vi "Actor Core.vi"(8 "error in":errorcluster, 11 "WebSocket Connection in":refnum<class "WebSocket Connection.lvclass">) -> (0 "error out":errorcluster, 3 "Actor out":refnum<class "Actor.lvclass">)   [LabVIEW 2021, in "WebSocket Actors.lvlib" / "WebSocket Connection.lvclass"]
doc: "(<B>Filename</B>: Actor Framework.lvlib:Actor.lvclass:Actor Core.vi)\n\nReceives messages to the actor, reacts to them, and initiates any error handling that may shut the actor down.\n\nDescendant classes may override this VI to append parallel tasks for the actor to complete while it handles messages. Overrides use the Call Parent Method node."
uses:
  WebSocket Connection.lvclass
  C:/Program Files/National Instruments/LabVIEW 2021/vi.lib/ActorFramework/Actor/Actor.lvclass
  <vilib>/ActorFramework/Actor/Actor.lvclass
  Abstract Messages/WebSocket Connection Handler Msg/properties/Connection Event.ctl
  Abstract Messages/WebSocket Connection Handler Msg/typedefs/Message Data.ctl
  <vilib>/ActorFramework/Message Enqueuer/Message Enqueuer.lvclass
  <vilib>/LS Instruments AG/LV-WebSockets/Data Format.ctl
  <vilib>/ActorFramework/Actor/Actor.lvclass/Actor.ctl
  <vilib>/ActorFramework/Message Enqueuer/Message Enqueuer.lvclass/Message Enqueuer.ctl
  WebSocket Connection.lvclass/WebSocket Connection.ctl
  Abstract Messages/WebSocket Connection Handler Msg/WebSocket Connection Handler Msg.lvclass/WebSocket Connection Handler Msg.ctl
  Connection Status.ctl
  <vilib>/ActorFramework/Report Error Msg/Report Error Msg.lvclass/Report Error Msg.ctl
  <vilib>/ActorFramework/Message Enqueuer/Init from Existing Queue.vi
  <vilib>/ActorFramework/Message Enqueuer/Enqueue.vi
  <vilib>/GPower/Error/Library/SplitAppended.vi
  <vilib>/GPower/Error/Library/AppendErrors.vi
  <vilib>/GPower/Error/Library/Append/AppendMulti.vi
  <vilib>/GPower/Error/Library/SubVIs/ExplanationToError.vi
  <vilib>/dlg_ctls.llb/Space Constant.vi
  Abstract Messages/WebSocket Connection Handler Msg/WebSocket Connection Handler Msg.lvclass
  C:/Program Files/National Instruments/LabVIEW 2021/vi.lib/ActorFramework/Message/Message.lvclass
  <vilib>/ActorFramework/Report Error Msg/Report Error Msg.lvclass
  <vilib>/ActorFramework/Stop Msg/Stop Msg.lvclass
  <vilib>/Utility/LVClass/Get LV Class Name.vi
  <resource>/AFDebug/Generate Trace for Message.vi
  <vilib>/ActorFramework/Message Priority Queue/Priority Enqueue.vi
  <vilib>/Utility/error.llb/Error Cluster From Error Code.vi
  <vilib>/Utility/error.llb/Trim Whitespace.vi
  <vilib>/Utility/error.llb/Error Code Database.vi
  <vilib>/GPower/Error/Library/Append/AppendSingle.vi
  <vilib>/ErrorRing/Error Ring.xnode
  WebSocket Connection Messages/Write Connection Status Msg/Write Connection Status Msg.lvclass
  <vilib>/LS Instruments AG/LV-WebSockets/LV WebSockets.lvlib
  <vilib>/GPower/Error/GPError.lvlib
  C:/Projects/WebSocket-Actor/WebSocket Actor/WebSocket Connection/WebSocket Connection.lvclass
  Keepalive Heartbeat Messages/Report Pong Msg/Report Pong Msg.lvclass
  <userlib>/_OpenG.lib/error/error.llb/openg_error.lvlib
panel:
  out "Received Data":string
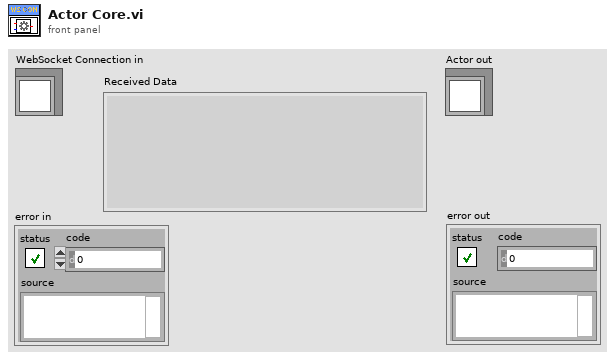
[diagram p1: front panel]
types:
  T1 = typedef "WebSocket Actors.lvlib/WebSocket Connection Handler Msg.lvclass/Message Data.ctl" = cluster{"Data":string, "Peer ID":string, "Connection Enqueuer":refnum<class "Message Enqueuer.lvclass">, "Data Format":T2}
  T2 = typedef "LV WebSockets.lvlib/Data Format.ctl" = enum16{"Text", "Binary"}
  T3 = typedef "WebSocket Actors.lvlib/WebSocket Connection Handler Msg.lvclass/Connection Event.ctl" = enum16{"On Connect", "On Message", "On Close", "On Drop"}
  T4 = typedef "WebSocket Actors.lvlib/WebSocket Connection.lvclass/Connection Status.ctl" = enum16{"Open", "Closed by Self", "Closed by Peer", "Dropped"}
  T5 = typedef "LV WebSockets.lvlib/Opcode.ctl" = enum8{"Continuation Frame", "Text Frame", "Binary Frame", "Reserved 3", "Reserved 4", "Reserved 5", "Reserved 6", "Reserved 7", "Connection Close", "Ping", "Pong", "Reserved B", "Reserved C", "Reserved D", "Reserved F"}
  T6 = typedef "LV WebSockets.lvlib/StatusCode.ctl" = u16
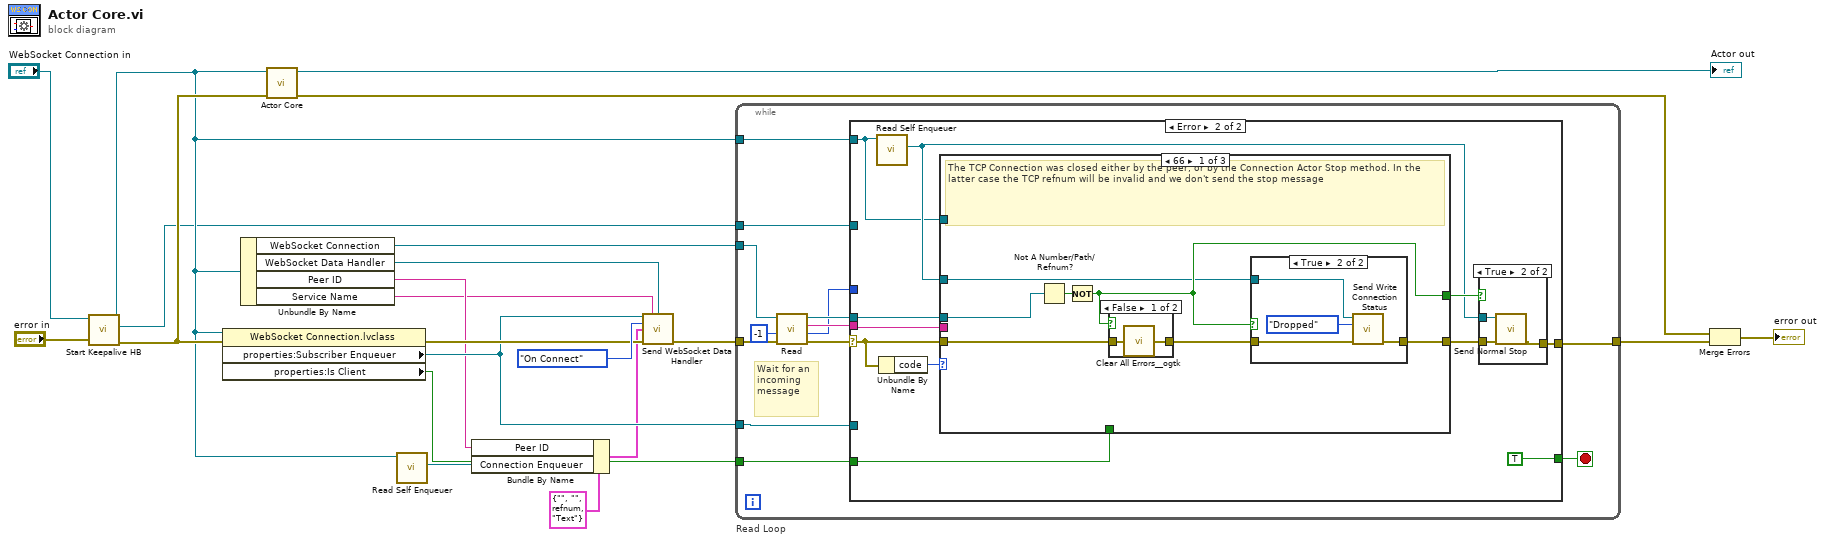
[diagram p0: block diagram]
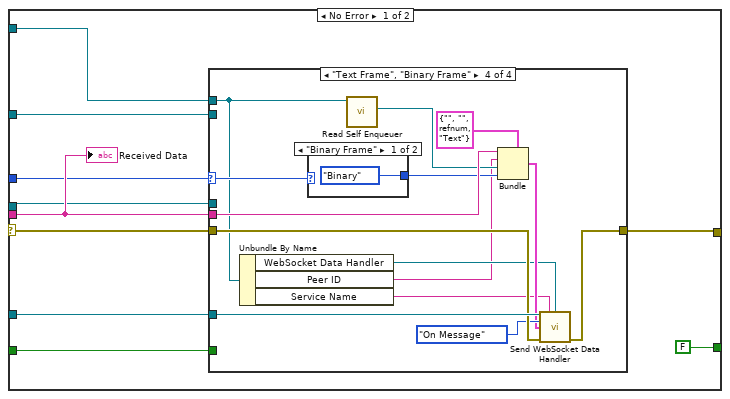
[diagram p2: hidden frame]
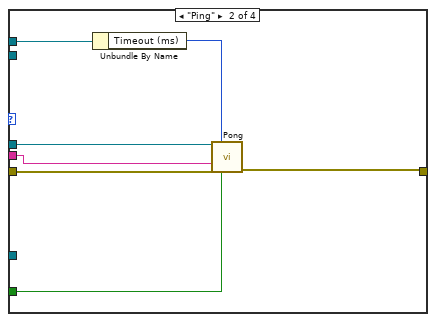
[diagram p4: hidden frame]
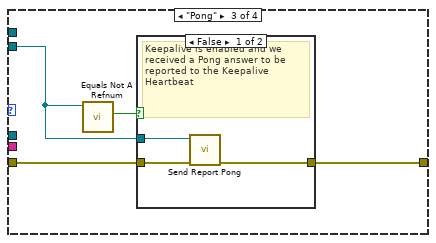
[diagram p5: hidden frame]
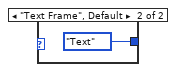
[diagram p7: hidden frame]
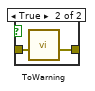
[diagram p10: hidden frame]
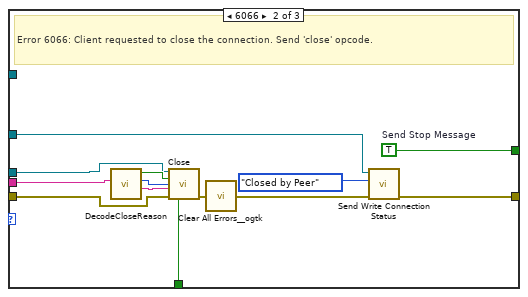
[diagram p11: hidden frame]
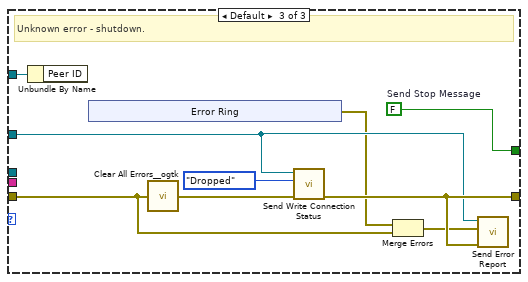
[diagram p12: hidden frame]
diagram:
  n1 = call "Start Keepalive HB.vi"("error in (no error)"="error in", "WebSocket Connection in"="WebSocket Connection in") -> ("error out"=w4:errorcluster, "Keepalive Heartbeat's Enqueuer"=w1:refnum<class "Message Enqueuer.lvclass">, "WebSocket Connection out"=w2:refnum<class "WebSocket Connection.lvclass">)  [unwired: 7 in]
  n2 = property class="WebSocket Connection.lvclass"(reference=w2, error in=w4) -> (error out=w13:errorcluster, "properties:Subscriber Enqueuer"=w12:refnum<class "Message Enqueuer.lvclass">, "properties:Is Client"=w11:bool)  [unwired: 1 out]
  n3 = Unbundle By Name(w2) -> ("WebSocket Connection"=w20:refnum<k5>, "WebSocket Data Handler"=w17:refnum<class "WebSocket Connection Handler Msg.lvclass">, "Peer ID"=w8:string, "Service Name"=w6:string)
  n4 = call-parent "Actor Core.vi"("error in"=w4, "Actor in"=w2) -> ("error out"=w21:errorcluster, "Actor out"=→"Actor out":refnum<class "Actor.lvclass">)  [unwired: 8 in]
  n5 = call <vilib>:"Read Self Enqueuer.vi"("Actor"=w2) -> ("Self Enqueuer"=w9:refnum<class "Message Enqueuer.lvclass">)  [unwired: 10 in]
  n6 = Bundle By Name(cluster=T1 {"Data"="", "Peer ID"="", "Connection Enqueuer"=refnum, "Data Format"=enum."Text"} ("Connection Message Data"), "Peer ID"=w8, "Connection Enqueuer"=w9) -> (w7:T1)
  n7 = call "Send WebSocket Data Handler.vi"("Message Enqueuer"=w12, "Service Name"=w6, "Message Type"=w17, "Connection Event"=Connection_Event."On Connect", "Connection Message Data"=w7, "error in (no error)"=w13) -> ("error out"=w15:errorcluster)  [unwired: 8 in, 1 out]
  n8 = while "Read Loop" {
    tunnel: w20 -> [w34]
    tunnel: [w27] -> w18
    tunnel: w15 -> [w30]
    tunnel: w12 -> [w28]
    tunnel: w2 -> [w26]
    tunnel: w11 -> [w25]
    tunnel: w1 -> [w23]
    stop <- w29 stop-if-true
    # "Wait for an incoming message"
    n9 = call <vilib>:"Read.vi"("error in (no error)"=w30, "timeout ms (5000)"=-1 ("timeout ms (25000)"), "WebSocket Connection in"=w34) -> ("error out"=w22:errorcluster, "Opcode out"=w24:T5, "Data"=w32:string, "WebSocket Connection out"=w31:refnum<k5>)  [unwired: 5 in]
    n10 = case shown="Error" w22 {
      selector: w22 -> [w42 w85]
      tunnel: w32 -> [w40 w79]
      tunnel: w31 -> [w37 w86]
      tunnel: [FALSE TRUE] -> w29
      tunnel: w28 -> [w43 _]
      tunnel: [w41 w83] -> w27
      tunnel: w26 -> [w39 w77]
      tunnel: w25 -> [w36 w80]
      tunnel: w24 -> [w38 _]
      tunnel: w23 -> [w35 _]
      frame No Error {
        n11 = case shown="\"Ping\"" w38 {
          selector: w38 -> [_ _ _ w67]
          tunnel: w43 -> [_ _ _ w74]
          tunnel: w42 -> [w45 w52 w55 w73]
          tunnel: [w45 w51 w54 w72] -> w41
          tunnel: w40 -> [_ w49 _ w69]
          tunnel: w39 -> [_ w48 _ w64]
          tunnel: w37 -> [_ w50 _ _]
          tunnel: w36 -> [_ w47 _ _]
          tunnel: w35 -> [_ _ w53 _]
          frame "Continuation Frame", Default {
          }
          frame "Ping" {
            n12 = Unbundle By Name(w48) -> ("Timeout (ms)"=w46:i32)
            n13 = call <vilib>:"Pong.vi"("WebSocket Connection in"=w50, "timeout ms (5000)"=w46, "Data"=w49, "error in (no error)"=w52, "Mask payload?"=w47) -> ("error out"=w51:errorcluster)  [unwired: 9 in, 1 out]
          }
          frame "Pong" {
            n14 = call <vilib>:"Equals Not A Refnum.vi"("Message Enqueuer"=w53) -> ("Not a refnum?"=w56:bool)  [unwired: 10 in]
            n15 = case shown="False" w56 {
              tunnel: w55 -> [w59 w60]
              tunnel: [w58 w60] -> w54
              tunnel: w53 -> [w57 _]
              frame False {
                # "Keepalive is enabled and we received a Pong answer to be reported to the Keepalive Heartbeat"
                n16 = call "Send Report Pong.vi"("error in (no error)"=w59, "Message Enqueuer in"=w57) -> ("error out"=w58:errorcluster)  [unwired: 8 in, 1 out]
              }
              frame True {
              }
            }
          }
          frame "Text Frame", "Binary Frame" {
            n17 = Unbundle By Name(w64) -> ("WebSocket Data Handler"=w63:refnum<class "WebSocket Connection Handler Msg.lvclass">, "Peer ID"=w62:string, "Service Name"=w61:string)
            n18 = case shown="\"Binary Frame\"" w67 {
              tunnel: [Data_Format."Binary" ("Data Format") Data_Format."Text" ("Data Format")] -> w66
              frame "Binary Frame" {
              }
              frame "Text Frame", Default {
              }
            }
            n19 = call <vilib>:"Read Self Enqueuer.vi"("Actor"=w64) -> ("Self Enqueuer"=w68:refnum<class "Message Enqueuer.lvclass">)  [unwired: 10 in]
            n20 = Bundle(cluster=T1 {"Data"="", "Peer ID"="", "Connection Enqueuer"=refnum, "Data Format"=enum."Text"} ("Connection Message Data"), "Data"=w69, "Peer ID"=w62, "Connection Enqueuer"=w68, "Data Format"=w66) -> (w65:T1)
            n21 = call "Send WebSocket Data Handler.vi"("Message Enqueuer"=w74, "Service Name"=w61, "Message Type"=w63, "Connection Event"=Connection_Event."On Message", "Connection Message Data"=w65, "error in (no error)"=w73) -> ("error out"=w72:errorcluster)  [unwired: 8 in, 1 out]
          }
        }
        "Received Data" <- w40
      }
      frame Error {
        n22 = call <vilib>:"Read Self Enqueuer.vi"("Actor"=w77) -> ("Self Enqueuer"=w78:refnum<class "Message Enqueuer.lvclass">)  [unwired: 10 in]
        n23 = Unbundle By Name(w85) -> ("code"=w87:i32)
        n24 = case shown="66" w87 {
          tunnel: w86 -> [w97 w114 _]
          tunnel: w85 -> [w98 w115 w124]
          tunnel: [w94 w110 w126] -> w84
          tunnel: [w93 w120 w129] -> w82
          tunnel: w80 -> [_ w113 _]
          tunnel: w79 -> [_ w112 _]
          tunnel: w78 -> [w92 w109 w125]
          tunnel: w77 -> [_ _ w123]
          frame 66 {
            # "The TCP Connection was closed either by the peer, or by the Connection Actor Stop method. In the latter case the TCP refnum will be invalid and we don't send the stop message"
            n25 = Not A Number/Path/Refnum?(number/path/refnum=w97) -> (NaN/Path/Refnum?=w96:bool)
            n26 = Not(x=w96) -> (.not. x?=w93:bool)
            n27 = case shown="False" w93 {
              tunnel: w98 -> [w105 w107]
              tunnel: [w104 w106] -> w95
              frame False {
                n28 = call <userlib>:"Clear All Errors__ogtk.vi"("Error In"=w105) -> ("Error Out"=w104:errorcluster)  [unwired: 3 in]
              }
              frame True {
                n29 = call <vilib>:"ToWarning.vi"("Error in"=w107) -> ("Warning out"=w106:errorcluster)  [unwired: 10 in]
              }
            }
            n30 = case shown="True" w93 {
              tunnel: w95 -> [w99 w103]
              tunnel: [w99 w102] -> w94
              tunnel: w92 -> [_ w100]
              frame False {
              }
              frame True {
                n31 = call "Send Write Connection Status.vi"("error in (no error)"=w103, "Connection Status"=Connection_Status."Dropped", "Message Enqueuer in"=w100) -> ("error out"=w102:errorcluster)  [unwired: 7 in, 1 out]
              }
            }
          }
          frame 6066 {
            w120 = TRUE  # Send Stop Message
            # "Error 6066: Client requested to close the connection. Send 'close' opcode."
            n32 = call <vilib>:"DecodeCloseReason.vi"("Data"=w112) -> ("Reason"=w117:string, "Status Code"=w119:T6, "Close Reason Given"=w118:bool)  [unwired: 8 in]
            n33 = call <vilib>:"Close.vi"("WebSocket Connection in"=w114, "Send Reason (F)"=w118, "Status Code"=w119, "Reason"=w117, "error in (no error)"=w115, "Mask payload?"=w113) -> ("error out"=w116:errorcluster)  [unwired: 8 in, 1 out]
            n34 = call <userlib>:"Clear All Errors__ogtk.vi"("Error In"=w116) -> ("Error Out"=w111:errorcluster)  [unwired: 3 in]
            n35 = call "Send Write Connection Status.vi"("error in (no error)"=w111, "Connection Status"=Connection_Status."Closed by Peer", "Message Enqueuer in"=w109) -> ("error out"=w110:errorcluster)  [unwired: 7 in, 1 out]
          }
          frame Default {
            w129 = FALSE  # Send Stop Message
            # "Unknown error - shutdown."
            n36 = Unbundle By Name(w123) -> ()  [unwired: 1 out]
            n37 = xnode "Error Ring"() -> ("error out"=w121:errorcluster)
            n38 = call <userlib>:"Clear All Errors__ogtk.vi"("Error In"=w124) -> ("Error Out"=w127:errorcluster)  [unwired: 3 in]
            n39 = call "Send Write Connection Status.vi"("error in (no error)"=w127, "Connection Status"=Connection_Status."Dropped", "Message Enqueuer in"=w125) -> ("error out"=w126:errorcluster)  [unwired: 7 in, 1 out]
            n40 = Merge Errors(w121, w124) -> (w122:errorcluster)
            n41 = call <vilib>:"Send Error Report.vi"("error in (no error)"=w126, "Error From Sender"=w122, "Message Enqueuer"=w125) -> ()  [unwired: 8 in, 1 out]
          }
        }
        n42 = case shown="True" w82 {
          tunnel: w84 -> [w88 w91]
          tunnel: w78 -> [_ w90]
          tunnel: [w88 w89] -> w83
          frame False {
          }
          frame True {
            n43 = call <vilib>:"Send Normal Stop.vi"("error in (no error)"=w91, "Message Enqueuer"=w90) -> ("error out"=w89:errorcluster)  [unwired: 9 in]
          }
        }
      }
    }
  }
  n44 = Merge Errors(w21, w18) -> (→"error out":errorcluster)
